vi "CaseStructure.vi"(8 "error in":errorcluster, 11 "reference":refnum<vi>) -> (0 "error out":errorcluster, 3 "CaseStructure out":refnum<class "CaseStructure.lvclass">)   [LabVIEW 2014, in "Raspberry Pi Compatible Compiler for LabVIEW.lvlib" / "CaseStructure.lvclass"]
uses:
  CaseStructure.lvclass
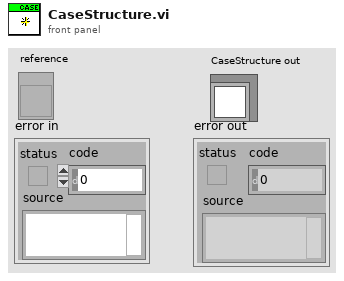
[diagram p1: front panel]
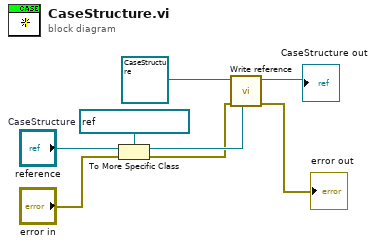
[diagram p0: block diagram]
diagram:
  w8 = refnum<vi> refnum  # CaseStructure
  n1 = To More Specific Class(target class=w8, reference="reference", error in="error in") -> (specific class reference=w4:refnum<vi>, error out=w2:errorcluster)
  n2 = call-dynamic "Write reference.vi"("reference"=w4, "error in"=w2, "GObject in"=refnum<class "CaseStructure.lvclass"> refnum ("CaseStructure out")) -> ("error out"=→"error out":errorcluster, "GObject out"=→"CaseStructure out":refnum<class "CaseStructure.lvclass">)  [unwired: 5 in]
